vi "StartUI.vi"(8 "error in (no error)":errorcluster, 11 "Execution in":refnum<data-value>) -> (0 "error out":errorcluster, 3 "Execution out":refnum<data-value>)   [LabVIEW 2015, in "Execution.lvclass"]
uses:
  Execution.lvclass
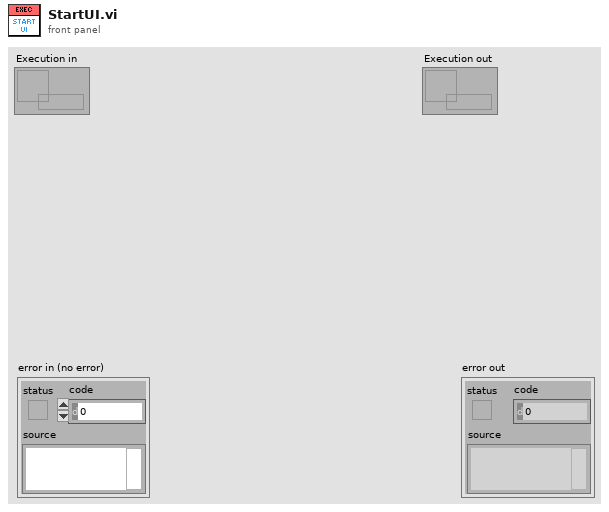
[diagram p1: front panel]
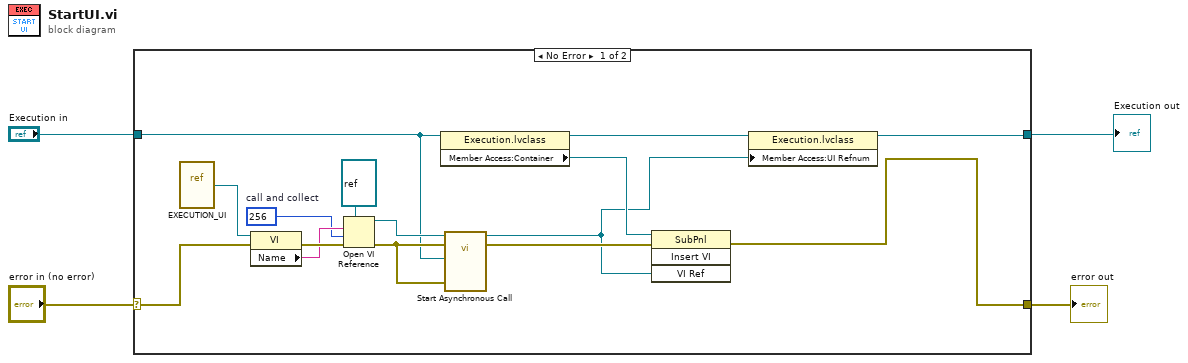
[diagram p0: block diagram]
diagram:
  n1 = case shown="No Error" "error in (no error)" {
    selector: "error in (no error)" -> [w11 w21]
    tunnel: [w10 w21] -> w3
    tunnel: [w6 w20] -> w1
    tunnel: "Execution in" -> [w9 w20]
    frame No Error {
      w13 = 256  # call and collect
      n2 = vi-ref "EXECUTION_UI.vi"() -> (w15:refnum<vi>)
      n3 = property class="VI"(reference=w15, error in=w11) -> (error out=w17:errorcluster, "Name"=w16:string)  [unwired: 1 out]
      n4 = Open VI Reference(type specifier VI Refnum (for type only)=refnum<vi> refnum ("VI Refnum"), vi path=w16, options=w13, error in (no error)=w17) -> (vi reference=w14:refnum<vi>, error out=w19:errorcluster)  [unwired: 2 in]
      n5 = property class="Execution.lvclass"(reference=w9) -> (reference out=w8:refnum<data-value>, "Member Access:Container"=w7:refnum<vi>)  [unwired: 1 in, 1 out]
      n6 = call-by-ref "Start Asynchronous Call"(reference=w14, error in=w19, 8:"error in (no error)"=w19, "Socket in"=w9) -> (reference out=w5:refnum<vi>, error out=w18:errorcluster)  [unwired: 8 in, 2 out]
      n7 = invoke class="SubPnl" method="Insert VI"(reference=w7, error in=w18, "VI Ref"=w5) -> (error out=w10:errorcluster)  [unwired: 1 in, 3 out]
      n8 = property class="Execution.lvclass"(reference=w8, "Member Access:UI Refnum"=w5) -> (reference out=w6:refnum<data-value>)  [unwired: 1 in, 1 out]
    }
    frame Error {
    }
  }
  "error out" <- w3
  "Execution out" <- w1
